vi "ISMBUS_GetLifeList.vi"(8 "Fehler (Eingang - kein Fehler)":errorcluster) -> (0 "Fehler (Ausgang)":errorcluster caption="error IO", 2 "Rückgabetyp":i32, 3 "ModuleArray":T1[](array[typedef]))   [LabVIEW 2013]
uses:
  ISMBUS_Module.ctl
  ISMBUS_Channel.ctl
  ISMBUS32.DLL
panel:
  out "ItemListItemSub1":i32
  out "ItemList":i32[](array[numeric])
  out "ItemCount":i32
  out "StructureID":i32
  out "AddArgument":i32
  out "MaxScanCount":i32
  out "ScanBaudrate":i32
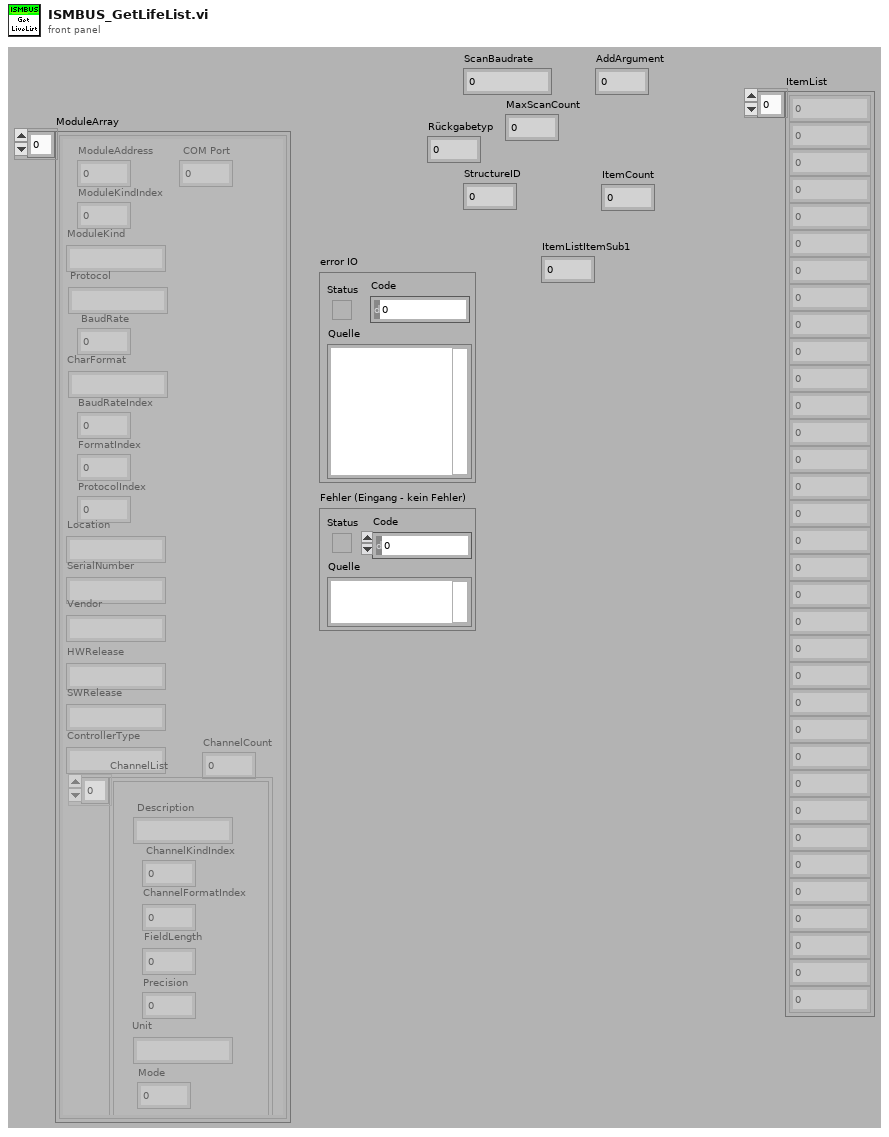
[diagram p1: front panel]
types:
  T1 = typedef "ISMBUS_Module.ctl" = cluster{"ModuleAddress":i32, "ModuleKindIndex":i32, "ModuleKind":string, " Protocol":string, " BaudRate":i32, "CharFormat":string, "BaudRateIndex":i32, "FormatIndex":i32, "ProtocolIndex":i32, "Location":string, "SerialNumber":string, "Vendor":string, "HWRelease":string, "SWRelease":string, "ControllerType":string, "ChannelList":T2[], "ChannelCount":i32, " COM Port":i32}
  T2 = typedef "ISMBUS_Channel.ctl" = cluster{" Description":string, " ChannelKindIndex":i32, "ChannelFormatIndex":i32, " FieldLength":i32, "Precision":i32, "Unit":string, "Mode":i32}
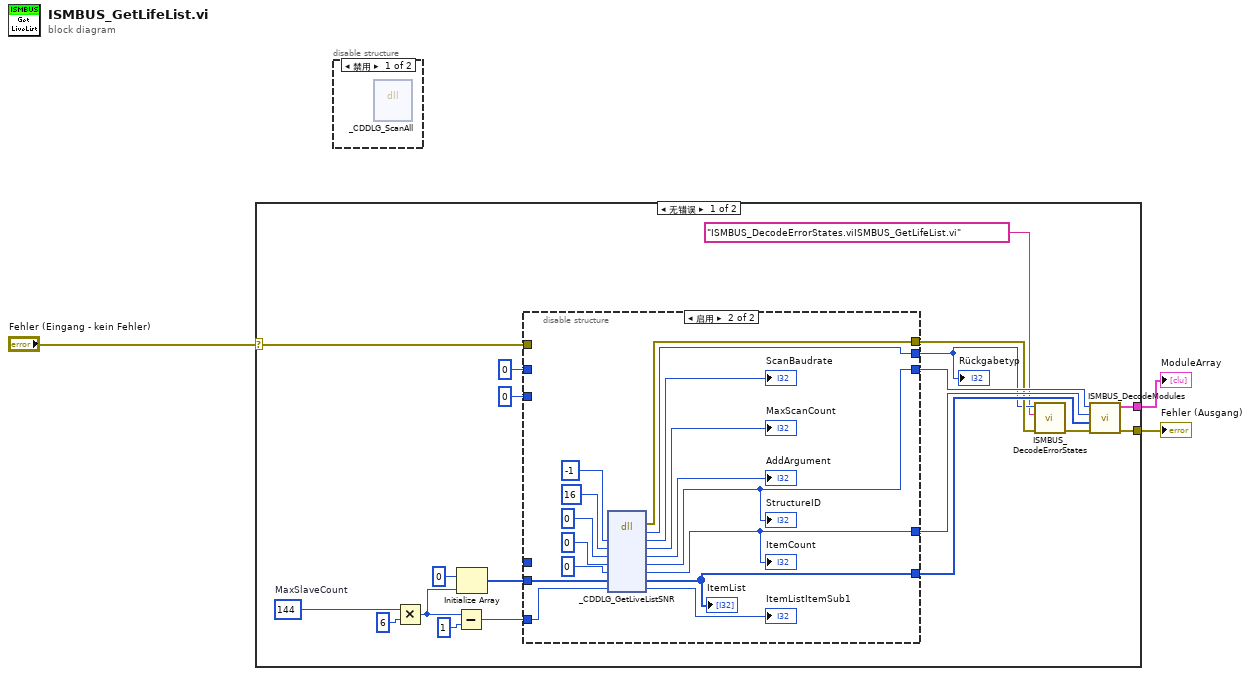
[diagram p0: block diagram]
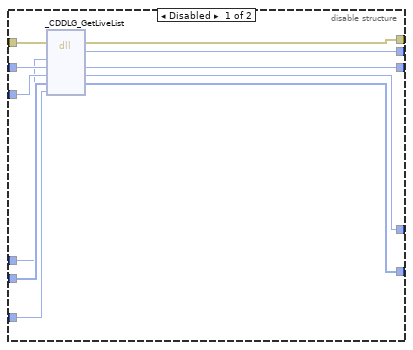
[diagram p3: hidden frame]
diagram:
  n1 = case shown="无错误" "Fehler (Eingang - kein Fehler)" {
    selector: "Fehler (Eingang - kein Fehler)" -> [w20 w50]
    tunnel: [w9 w50] -> w1
    tunnel: [w4 _] -> w2
    frame No Error {
      w15 = 144  # MaxSlaveCount
      n2 = Multiply(x=w15, y=6) -> (x*y=w13:i32)
      n3 = Subtract(x=w13, y=1) -> (x-y=w10:i32)
      n4 = Initialize Array(0 ("StructureID"), w13) -> (w11:i32[])
      n5 = disable-structure shown="启用" {
        disable-tunnel: 0 ("ItemCount") -> [w33 _]
        disable-tunnel: 0 ("StructureID") -> [w32 _]
        disable-tunnel: w20 -> [w31 _]
        disable-tunnel: [w30 w38] -> w19
        disable-tunnel: [w29 w39] -> w18
        disable-tunnel: [w28 w40] -> w17
        disable-tunnel: w11 -> [w27 w45]
        disable-tunnel: w10 -> [w26 w44]
        disable-tunnel: [w25 w41] -> w8
        disable-tunnel: [w24 w42] -> w7
        disable-tunnel: _ -> [w23 _]
        frame Disabled {
          n6 = dll-call lib="ISMBUS32.DLL" fn="_CDDLG_GetLiveList"(error in=w31, "ComPort"=w23, "StructureID"=w32, "ItemCount"=w33, "ArrItemList"=w27, "ItemListItemSub1"=w26) -> (error out=w25:errorcluster, "Rückgabetyp"=w24:i32, "StructureID"=w30:i32, "ItemCount"=w29:i32, "ArrItemList"=w28:i32[])  [unwired: 4 in, 1 out]
        }
        frame Enabled {
          n7 = dll-call lib="ISMBUS32.DLL" fn="_CDDLG_GetLiveListSNR"("ScanBaudrate"=-1, "MaxScanCount"=16, "AddArgument"=0, "StructureID"=0, "ItemCount"=0, "ItemList"=w45, "ItemListItemSub1"=w44) -> (error out=w41:errorcluster, "Rückgabetyp"=w42:i32, "ScanBaudrate"=→"ScanBaudrate":i32, "MaxScanCount"=→"MaxScanCount":i32, "AddArgument"=→"AddArgument":i32, "StructureID"=w38:i32, "ItemCount"=w39:i32, "ItemList"=w40:i32[], "ItemListItemSub1"=→"ItemListItemSub1":i32)  [unwired: 3 in, 1 out]
          "StructureID" <- w38
          "ItemCount" <- w39
          "ItemList" <- w40
        }
      }
      "Rückgabetyp" <- w7
      n8 = call "ISMBUS_DecodeErrorStates.vi"("Fehler (Eingang - kein Fehler)"=w8, "Location"="ISMBUS_DecodeErrorStates.viISMBUS_GetLifeList.vi", "ISMBUS_Error State"=w7) -> ("Fehler (Ausgang)"=w6:errorcluster)  [unwired: 8 out]
      n9 = call "ISMBUS_DecodeModules.vi"("error in"=w6, "Array"=w17, "ItemsCount"=w18, "Stricture ID"=w19) -> ("error out"=w9:errorcluster, "ModuleArray"=w4:T1[])  [unwired: 1 in, 5 out]
    }
    frame Error {
    }
  }
  "ModuleArray" <- w2
  "Fehler (Ausgang)" <- w1
  n10 = disable-structure shown="禁用" {
    frame Disabled {
      n11 = dll-call lib="ISMBUS32.DLL" fn="_CDDLG_ScanAll"() -> ()  [unwired: 5 in, 5 out]
    }
    frame Enabled {
    }
  }
